vi "SysDef.Globals.vi"() -> ()   [LabVIEW 2024, in "Advanced System Definition.lvlib"]
uses:
  SysDef API/Advanced System Definition.lvlib
panel:
  in  "Version":string="1.0.0"
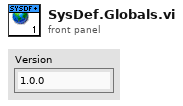
[diagram p1: front panel]
diagram:
